vi "api_mqttConnect.vi"(8 "error in (no error)":errorcluster, 11 "MQTT In":refnum<class "mqtt.lvclass">) -> (0 "error out":errorcluster, 1 "sessionPresent":bool, 2 "success":bool, 3 "MQTT Out":refnum<class "mqtt.lvclass">, 4 "connStatus":T1=enum."Connection refused: not authorized")   [LabVIEW 2020, in "mqtt.lvclass"]
uses:
  mqtt.lvclass
  mqttTypedef/mqttConnectionStatus.ctl
  mqttCmd/mqttCmdConnect/ConnectMqttMsg.lvclass
  C:/Projects/Libraries/Gore SM 2020/mqtt-LabVIEW/src/class/mqtt/mqttCmd/BaseMqttMsg.lvclass
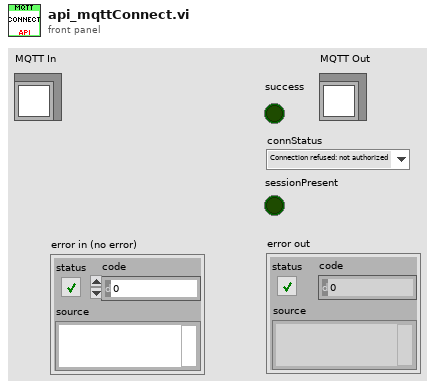
[diagram p1: front panel]
types:
  T1 = typedef "mqtt.lvclass/mqttConnectionStatus.ctl" = enum16{"Connection accepted", "Connection refused: unacceptable protocol version", "Connection refused: identifier rejected", "Connection refused: Server unavailable", "Connection refused: bad user name or password", "Connection refused: not authorized"}
  T2 = typedef "mqttConnectionStatus.ctl" = enum16{"Connection accepted", "Connection refused: unacceptable protocol version", "Connection refused: identifier rejected", "Connection refused: Server unavailable", "Connection refused: bad user name or password", "Connection refused: not authorized"}
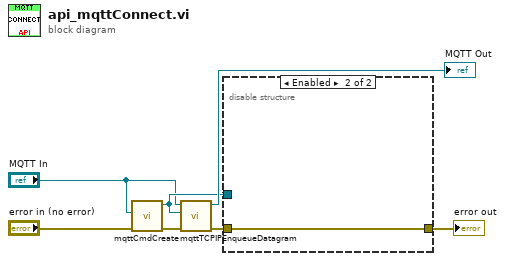
[diagram p0: block diagram]
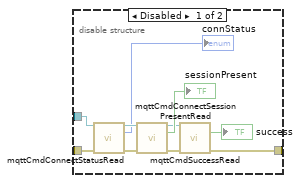
[diagram p2: hidden frame]
diagram:
  n1 = call "mqttCmdCreate.vi"("error in (no error)"="error in (no error)", "mqtt instance"="MQTT In") -> ("error out"=w3:errorcluster, "mqttCmdConnect out"=w2:refnum<class "ConnectMqttMsg.lvclass">)  [unwired: 8 in]
  n2 = call "mqttTCPIPEnqueueDatagram.vi"("error in (no error)"=w3, "mqttCmd"=w2, "mqtt in"="MQTT In") -> ("error out"=w5:errorcluster, "mqtt out"=→"MQTT Out":refnum<class "mqtt.lvclass">)  [unwired: 7 in]
  n3 = disable-structure shown="Enabled" {
    disable-tunnel: [w12 w18] -> w7
    disable-tunnel: w2 -> [w9 _]
    disable-tunnel: w5 -> [w8 w18]
    frame Disabled {
      n4 = call "mqttCmdConnectStatusRead.vi"("mqttConnect in"=w9, "error in (no error)"=w8) -> ("mqttConnect out"=w16:refnum<class "mqttCmdConnect.lvclass">, "connStatus"=→"connStatus":T2, "error out"=w17:errorcluster)  [unwired: 11 in]
      n5 = call "mqttCmdConnectSessionPresentRead.vi"("mqttConnect in"=w16, "error in (no error)"=w17) -> ("mqttConnect out"=w11:refnum<class "mqttCmdConnect.lvclass">, "sessionPresent"=→"sessionPresent":bool, "error out"=w13:errorcluster)  [unwired: 11 in]
      n6 = call "mqttCmdSuccessRead.vi"("mqttBrokerCommand in"=w11, "error in (no error)"=w13) -> ("success"=→"success":bool, "error out"=w12:errorcluster)  [unwired: 11 in, 1 out]
    }
    frame Enabled {
    }
  }
  "error out" <- w7
